vi "Get Data BY Serial Data.vi"(9 "HEAD":string, 10 "Data in":u8[](array[numeric]) format="%x") -> (1 "Data":string, 2 "Data Type":string)   [LabVIEW 2013]
panel:
  out "Data Array":u8[](array[numeric]) format="%x"
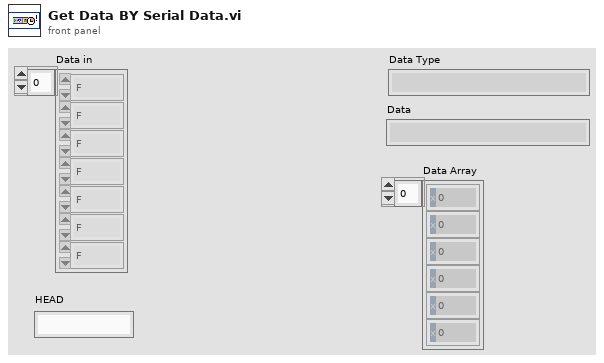
[diagram p1: front panel]
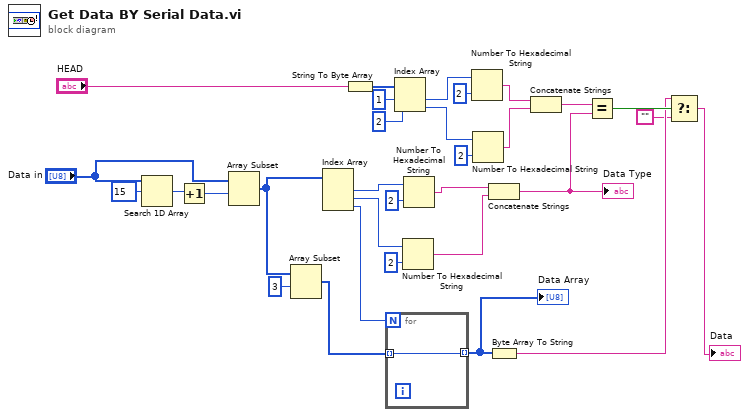
[diagram p0: block diagram]
diagram:
  n1 = Search 1D Array(1D array="Data in", element=u8 15 ("元素")) -> (index of element=w28:i32)  [unwired: 1 in]
  n2 = Increment(x=w28) -> (x+1=w26:i32)
  n3 = Array Subset(array="Data in", index=w26) -> (w20:u8[])  [unwired: 1 in]
  n4 = Array Subset(array=w20, index=3 ("索引")) -> (w18:u8[])  [unwired: 1 in]
  n5 = Index Array(array=w20) -> (element #1=w30:u8, element #2=w24:u8, element #3=w21:u8)  [unwired: 3 in]
  n6 = String To Byte Array(string="HEAD") -> (unsigned byte array=w15:u8[])
  n7 = for {
    N: w21 -> [_]
    tunnel: w18 -> [w32] mode=indexing
    tunnel: [w32] -> w17 mode=indexing
  }
  "Data Array" <- w17
  n8 = Index Array(array=w15, index #1=1 ("索引"), index #2=2 ("索引")) -> (element #1=w10:u8, element #2=w9:u8)
  n9 = Number To Hexadecimal String(1:i16 2 ("宽度(-)"), 2:w24) -> (0:w22:string)
  n10 = Number To Hexadecimal String(1:i16 2 ("宽度(-)"), 2:w30) -> (0:w23:string)
  n11 = Number To Hexadecimal String(1:i16 2 ("宽度(-)"), 2:w10) -> (0:w8:string)
  n12 = Number To Hexadecimal String(1:i16 2 ("宽度(-)"), 2:w9) -> (0:w7:string)
  n13 = Concatenate Strings(w23, w22) -> (w5:string)
  "Data Type" <- w5
  n14 = Byte Array To String(unsigned byte array=w17) -> (string=w3:string)
  n15 = Concatenate Strings(w8, w7) -> (w6:string)
  n16 = Equal?(x=w6, y=w5) -> (x = y?=w4:bool)
  n17 = Select(t=w3, s=w4, f="") -> (s? t:f=→"Data":string)
